vi "Flatten Tree.vi"(8 "error in":errorcluster, 10 "Flat Tree In":refnum<data-value>, 11 "Branch In":refnum<data-value>) -> (0 "error out":errorcluster, 2 "Flat Tree Out":refnum<data-value>, 3 "Branch Out":refnum<data-value>)   [LabVIEW 2019, in "Tree.lvclass"]
uses:
  Tree.lvclass
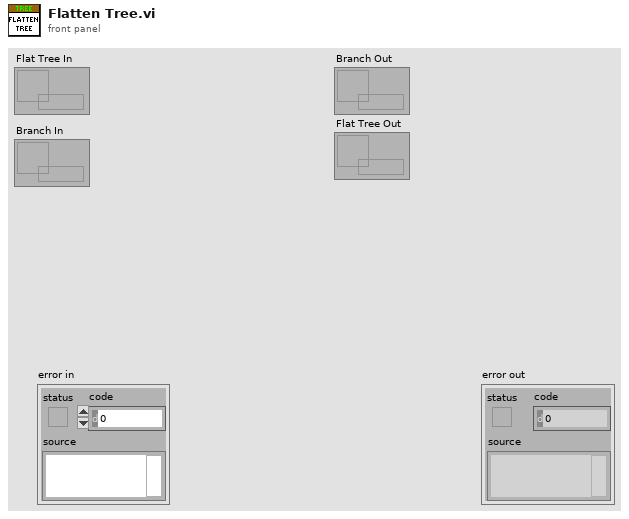
[diagram p1: front panel]
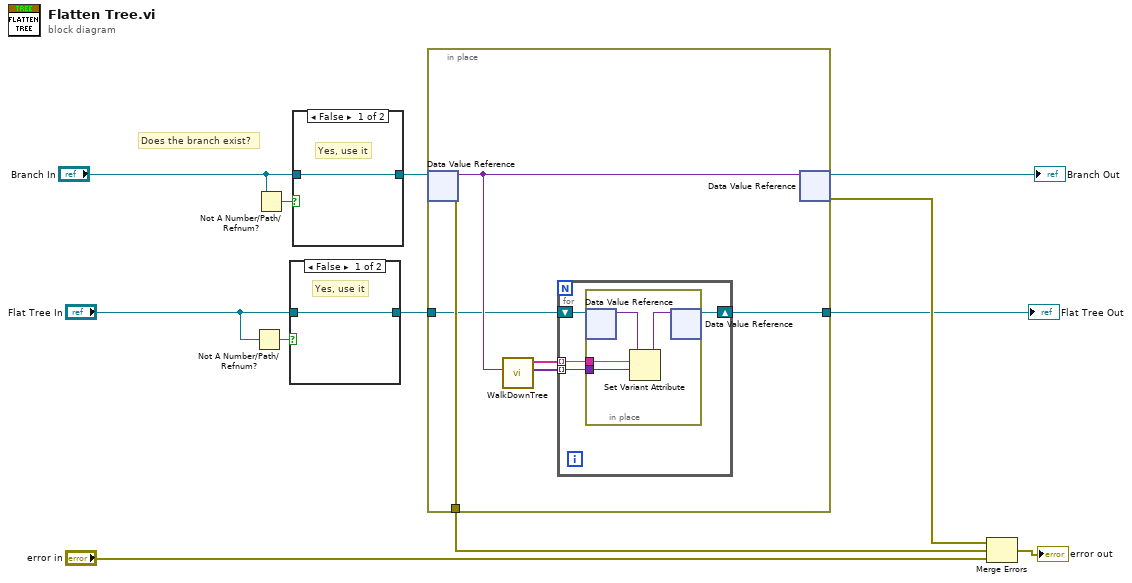
[diagram p0: block diagram]
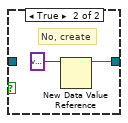
[diagram p2: hidden frame]
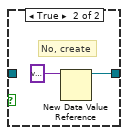
[diagram p3: hidden frame]
diagram:
  # "Does the branch exist?"
  n1 = Not A Number/Path/Refnum?(number/path/refnum="Flat Tree In") -> (NaN/Path/Refnum?=w3:bool)
  n2 = Not A Number/Path/Refnum?(number/path/refnum="Branch In") -> (NaN/Path/Refnum?=w8:bool)
  n3 = case shown="False" w3 {
    tunnel: [w13 w15] -> w2
    tunnel: "Flat Tree In" -> [w13 _]
    frame False {
      # "Yes, use it"
    }
    frame True {
      # "No, create"
      n4 = New Data Value Reference(data value=variant) -> (data value reference=w15:refnum<data-value>)  [unwired: 1 in, 1 out]
    }
  }
  n5 = case shown="False" w8 {
    tunnel: [w16 w18] -> w7
    tunnel: "Branch In" -> [w16 _]
    frame False {
      # "Yes, use it"
    }
    frame True {
      # "No, create"
      n6 = New Data Value Reference(data value=variant) -> (data value reference=w18:refnum<data-value>)  [unwired: 1 in, 1 out]
    }
  }
  n7 = in-place {
    in-place-border: [w24] -> w9
    in-place-border: w2 -> [w20]
    in-place-border: [w19] -> w1
    n8 = in-place-dvr #1(w7) -> (w23:variant, w24:errorcluster)
    n9 = call "WalkDownTree.vi"("Node In"=w23) -> ("Nodes Out"=w21:variant[], "Names"=w22:string[])  [unwired: 8 in, 1 out]
    n10 = for {
      tunnel: w22 -> [w28] mode=indexing
      tunnel: w21 -> [w26] mode=indexing
      shift-right: [w25] -> w19
      shift-left: w20 -> [w27]
      n11 = in-place {
        in-place-border: w28 -> [w31]
        in-place-border: w26 -> [w30]
        n12 = in-place-dvr #2(w27) -> (w32:variant)  [unwired: 1 out]
        n13 = Set Variant Attribute(Variant=w32, name=w31, value=w30) -> (Variant out=w29:variant)  [unwired: 1 in, 2 out]
        n14 = in-place-dvr #2(w29) -> (w25:refnum<data-value>)  [unwired: 1 out]
      }
    }
    n15 = in-place-dvr #1(w23) -> (→"Branch Out":refnum<data-value>, w10:errorcluster)
  }
  "Flat Tree Out" <- w1
  n16 = Merge Errors(w10, w9, "error in") -> (→"error out":errorcluster)
